vi "leer.vi"() -> ()   [LabVIEW 2016]
panel:
  out "XY Graph 3":cluster{dbl[], dbl[]}(graph)
  in  "file path (use dialog) 3":path
  out "XY Graph 2":cluster{dbl[], dbl[]}(graph)
  in  "file path (use dialog) 2":path
  out "XY Graph":cluster{dbl[], dbl[]}(graph)
  in  "file path (use dialog)":path
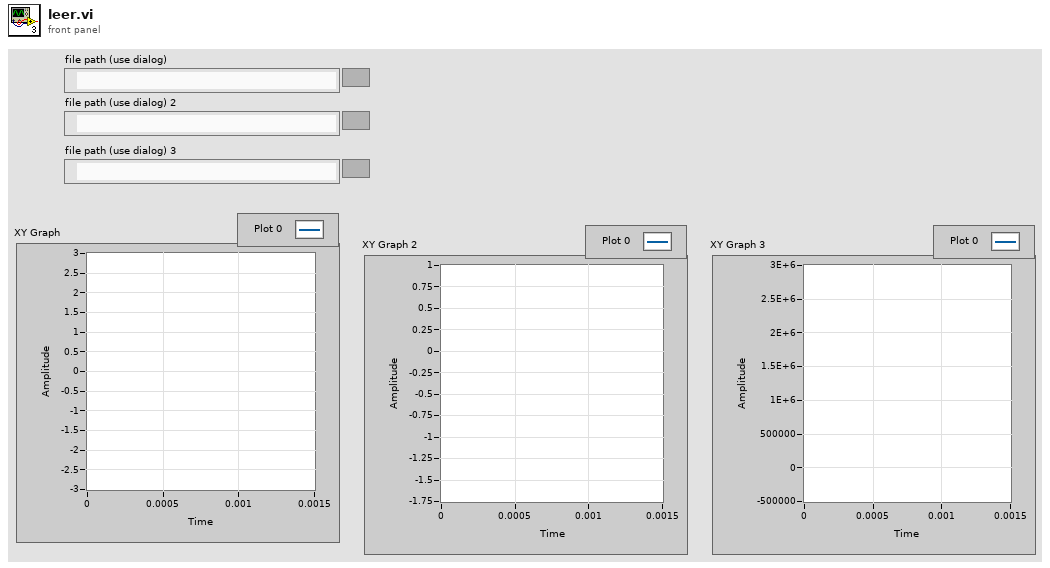
[diagram p1: front panel]
types:
  T1 = enum16{"open", "replace", "create", "open or create", "replace or create", "replace or create with confirmation"}
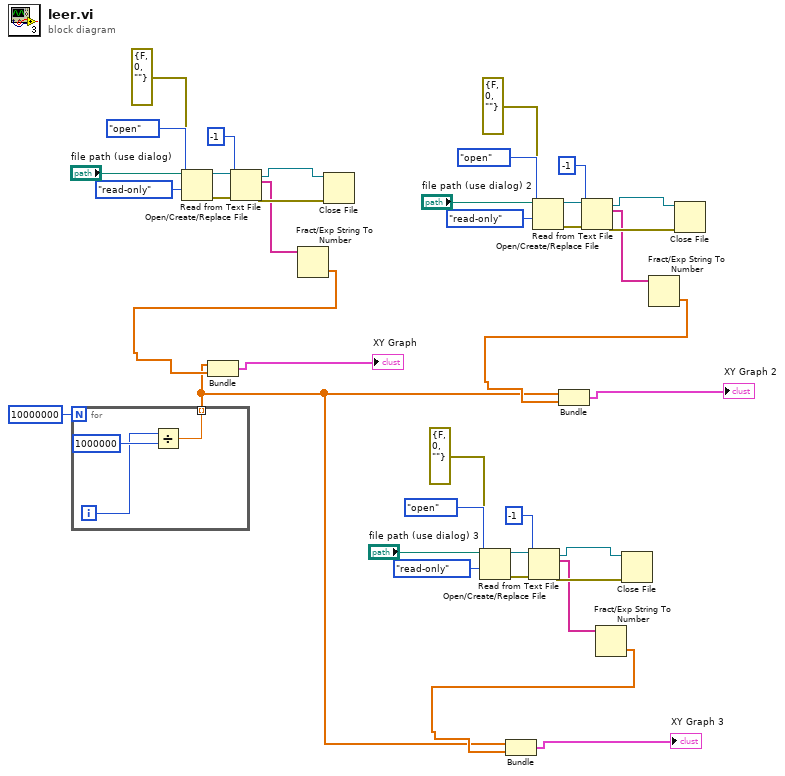
[diagram p0: block diagram]
diagram:
  n1 = for {
    N: 10000000 -> [_]
    tunnel: [w39] -> w1 mode=indexing
    i -> [w40]
    n2 = Divide(x=w40, y=u32 1000000) -> (x/y=w39:dbl)
  }
  n3 = Open/Create/Replace File(file path (use dialog)="file path (use dialog)", error in=errorcluster {"status"=FALSE, "code"=0, "source"=""}, operation (0:open)=T1."open", access (0:read/write)=enum16{"read/write", "read-only", "write-only"}."read-only") -> (refnum out=w34:refnum<file>, error out=w35:errorcluster)  [unwired: 2 in, 1 out]
  n4 = Read from Text File(file (use dialog)=w34, count=-1, error in=w35) -> (refnum out=w31:refnum<file>, text=w29:string[], error out=w32:errorcluster)  [unwired: 1 in, 1 out]
  n5 = Fract/Exp String To Number(string=w29) -> (number=w26:dbl[])  [unwired: 3 in, 1 out]
  n6 = Bundle(w1, w26) -> (→"XY Graph":cluster{dbl[], dbl[]})  [unwired: 1 in]
  n7 = Close File(refnum=w31, error in=w32) -> ()  [unwired: 2 out]
  n8 = Open/Create/Replace File(file path (use dialog)="file path (use dialog) 3", error in=errorcluster {"status"=FALSE, "code"=0, "source"=""}, operation (0:open)=T1."open", access (0:read/write)=enum16{"read/write", "read-only", "write-only"}."read-only") -> (refnum out=w9:refnum<file>, error out=w10:errorcluster)  [unwired: 2 in, 1 out]
  n9 = Read from Text File(file (use dialog)=w9, count=-1, error in=w10) -> (refnum out=w6:refnum<file>, text=w4:string[], error out=w7:errorcluster)  [unwired: 1 in, 1 out]
  n10 = Open/Create/Replace File(file path (use dialog)="file path (use dialog) 2", error in=errorcluster {"status"=FALSE, "code"=0, "source"=""}, operation (0:open)=T1."open", access (0:read/write)=enum16{"read/write", "read-only", "write-only"}."read-only") -> (refnum out=w21:refnum<file>, error out=w22:errorcluster)  [unwired: 2 in, 1 out]
  n11 = Read from Text File(file (use dialog)=w21, count=-1, error in=w22) -> (refnum out=w18:refnum<file>, text=w16:string[], error out=w19:errorcluster)  [unwired: 1 in, 1 out]
  n12 = Fract/Exp String To Number(string=w4) -> (number=w2:dbl[])  [unwired: 3 in, 1 out]
  n13 = Bundle(w1, w2) -> (→"XY Graph 3":cluster{dbl[], dbl[]})  [unwired: 1 in]
  n14 = Close File(refnum=w6, error in=w7) -> ()  [unwired: 2 out]
  n15 = Fract/Exp String To Number(string=w16) -> (number=w14:dbl[])  [unwired: 3 in, 1 out]
  n16 = Bundle(w1, w14) -> (→"XY Graph 2":cluster{dbl[], dbl[]})  [unwired: 1 in]
  n17 = Close File(refnum=w18, error in=w19) -> ()  [unwired: 2 out]
